vi "Test various FSW functions.vi"() -> ()   [LabVIEW 2020]
uses:
  SA-FSW.lvclass
  C:/Sandbox/RF Bench/Source Code/WiSpry Test Framework/Instruments/Spectrum Analyzer/Spectrum Analyzer.lvclass
  Controls/Marker Search.ctl
  Spectrum Analyzer.lvclass
  C:/Sandbox/RF Bench/Source Code/WiSpry Test Framework/Instruments/Instrument.lvclass
  Instrument.lvclass/Instrument.ctl
  Instrument.lvclass
panel:
  out "Min Freq":dbl
  out "Max freq":dbl
  out "min value":dbl
  out "max value":dbl
  out "XY Graph":cluster{"Frequency/Time":dbl[], "Level":dbl[]}(graph)
  out "Marker Level":dbl
  out "Marker Frequency/Time":dbl
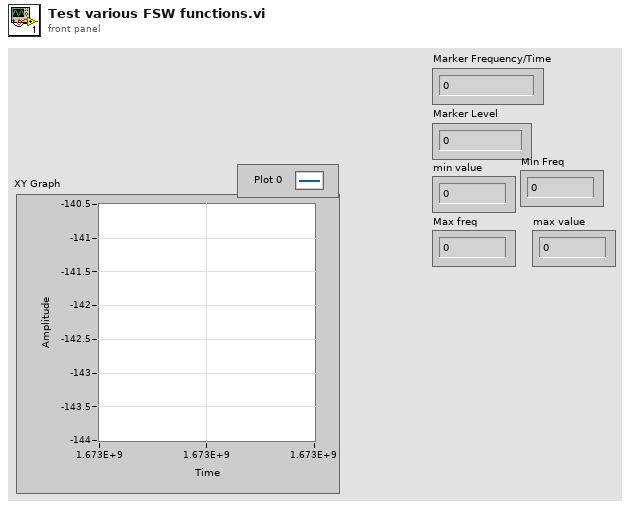
[diagram p1: front panel]
types:
  T1 = enum16{"Auto Peak", "Negative Peak", "Positive Peak", "Quasipeak", "Sample", "RMS", "Average", "CISPR Average", "CISPR RMS"}
  T2 = typedef "Spectrum Analyzer.lvclass/Marker Search.ctl" = enum16{"Maximum Peak", "Maximum Next", "Maximum Right", "Maximum Left", "Minimum Peak", "Minimum Next", "Minimum Right", "Minimum Left"}
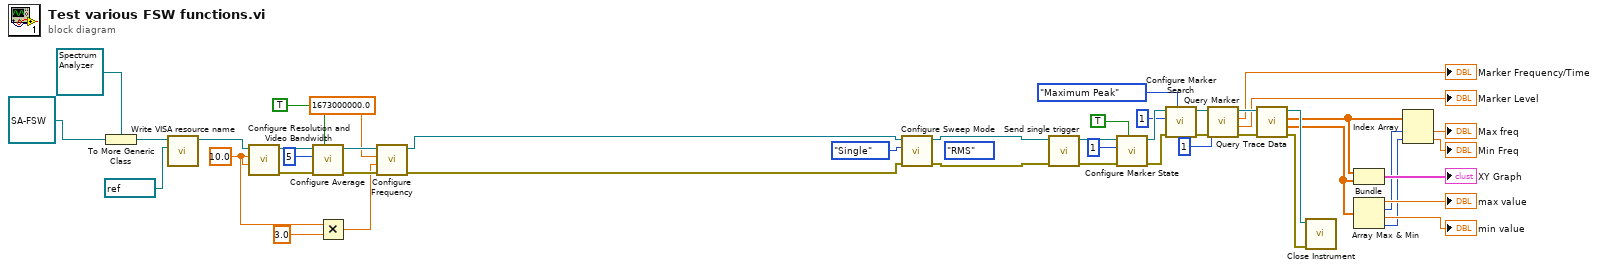
[diagram p0: block diagram]
diagram:
  w6 = 10.0 ("RBW [Hz]")
  (unwired) T1."RMS" ("Detector Mode")
  n1 = To More Generic Class(target class=refnum<class "Spectrum Analyzer.lvclass"> refnum ("Spectrum Analyzer.lvclass"), reference=refnum<class "SA-FSW.lvclass"> refnum ("SA-FSW.lvclass")) -> (generic class reference=w2:refnum<class "Spectrum Analyzer.lvclass">)
  n2 = call "Write VISA resource name.vi"("VISA resource name"=refnum<visa-resource-name> "FSW", "Instrument in"=w2) -> ("Instrument out"=w15:refnum<class "Spectrum Analyzer.lvclass">)  [unwired: 9 in]
  n3 = call-dynamic "Configure Resolution and Video Bandwidth.vi"("VBW [Hz]"=w6, "RBW [Hz]"=w6, "Spectrum Analyzer in"=w15) -> ("error out"=w11:errorcluster, "Spectrum Analyzer out"=w14:refnum<class "Spectrum Analyzer.lvclass">)  [unwired: 7 in]
  n4 = call-dynamic "Configure Average.vi"("Average On (F)"=TRUE, "error in (no error)"=w11, "Average"=u32 5, "Spectrum Analyzer in"=w14) -> ("error out"=w9:errorcluster, "Spectrum Analyzer out"=w10:refnum<class "Spectrum Analyzer.lvclass">)  [unwired: 6 in]
  n5 = Multiply(x=w6, y=3.0) -> (x*y=w7:dbl)
  n6 = call-dynamic "Configure Frequency.vi"("error in (no error)"=w9, "Span/Stop Frequency [Hz]"=w7, "Center/Start Frequency [Hz]"=1673000000.0, "Spectrum Analyzer in"=w10) -> ("error out"=w4:errorcluster, "Spectrum Analyzer out"=w3:refnum<class "Spectrum Analyzer.lvclass">)  [unwired: 6 in]
  n7 = call-dynamic "Configure Sweep Mode.vi"("error in (no error)"=w4, "Sweep Mode"=enum16{"Continuous", "Single"}."Single", "Spectrum Analyzer in"=w3) -> ("error out"=w19:errorcluster, "Spectrum Analyzer out"=w20:refnum<class "Spectrum Analyzer.lvclass">)  [unwired: 7 in]
  n8 = call-dynamic "Send single trigger.vi"("error in (no error)"=w19, "Spectrum Analyzer in"=w20) -> ("error out"=w44:errorcluster, "Spectrum Analyzer out"=w43:refnum<class "Spectrum Analyzer.lvclass">)  [unwired: 8 in]
  n9 = call-dynamic "Configure Marker State.vi"("Maker On (F)"=TRUE, "error in (no error)"=w44, "Marker Number (1)"=u32 1, "Spectrum Analyzer in"=w43) -> ("error out"=w41:errorcluster, "Spectrum Analyzer out"=w40:refnum<class "Spectrum Analyzer.lvclass">)  [unwired: 6 in]
  n10 = call-dynamic "Configure Marker Search.vi"("Marker Search (Max Peak)"=Marker_Search."Maximum Peak", "error in (no error)"=w41, "Marker Number (1)"=u32 1, "Spectrum Analyzer in"=w40) -> ("error out"=w38:errorcluster, "Spectrum Analyzer out"=w37:refnum<class "Spectrum Analyzer.lvclass">)  [unwired: 6 in]
  n11 = call-dynamic "Query Marker.vi"("error in (no error)"=w38, "Marker Number (1)"=u32 1, "Spectrum Analyzer in"=w37) -> ("error out"=w35:errorcluster, "Marker Level"=→"Marker Level":dbl, "Marker Frequency/Time"=→"Marker Frequency/Time":dbl, "Spectrum Analyzer out"=w36:refnum<class "Spectrum Analyzer.lvclass">)  [unwired: 5 in]
  n12 = call-dynamic "Query Trace Data.vi"("error in (no error)"=w35, "Spectrum Analyzer in"=w36) -> ("error out"=w30:errorcluster, "Level"=w29:dbl[], "Frequency/Time"=w26:dbl[], "Spectrum Analyzer out"=w31:refnum<class "Spectrum Analyzer.lvclass">)  [unwired: 6 in]
  n13 = call-dynamic "Close Instrument.vi"("error in (no error)"=w30, "Instrument in"=w31) -> ()  [unwired: 8 in, 2 out]
  n14 = Bundle("Frequency/Time"=w26, "Level"=w29) -> (→"XY Graph":cluster{"Frequency/Time":dbl[], "Level":dbl[]})  [unwired: 1 in]
  n15 = Array Max & Min(array=w29) -> (max value=→"max value":dbl, max index (indices)=w25:i32, min value=→"min value":dbl, min index (indices)=w24:i32)
  n16 = Index Array(array=w26, index #1=w25, index #2=w24) -> (element #1=→"Max freq":dbl, element #2=→"Min Freq":dbl)
